vi "Save Configuration Settings to XML.vi"(8 "error in (no error)":errorcluster, 11 "User Configuration":T1={"Hardware Configuration"={"HW Refnum <Replace Me>"="", "Signal Type <Replace Me>"=enum."Sine Wave"}, "Analysis Configuration"={"Statistics"=TRUE}, "New Data Behavior"=enum."Replace"}) -> (0 "error out":errorcluster)   [LabVIEW 2012]
doc: "Saves the user-specified configuration data to an XML file. This is used to remember settings between executions."
uses:
  controls/User Specified Data.ctl
  controls/HW Configuration.ctl
  controls/Simulated Signal Type.ctl
  controls/Analysis Configuration.ctl
  controls/New Data Behavior.ctl
  <vilib>/Utility/xml.llb/Write to XML File(string).vi
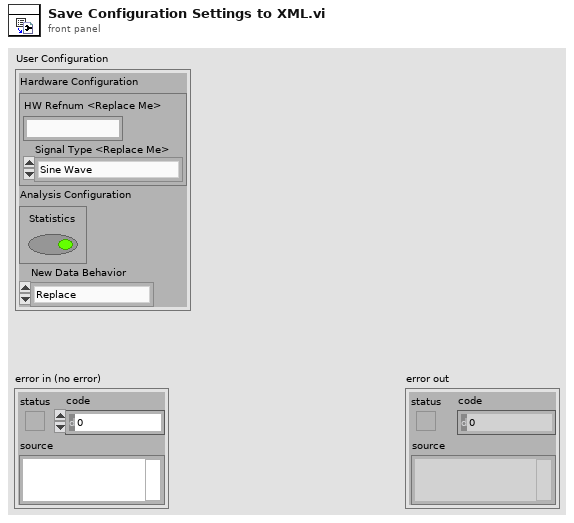
[diagram p1: front panel]
types:
  T1 = typedef "User Specified Data.ctl" = cluster{"Hardware Configuration":T2, "Analysis Configuration":T4, "New Data Behavior":T5}
  T2 = typedef "HW Configuration.ctl" = cluster{"HW Refnum <Replace Me>":string, "Signal Type <Replace Me>":T3}
  T3 = typedef "Simulated Signal Type.ctl" = enum16{"Sine Wave", "Square Wave"}
  T4 = typedef "Analysis Configuration.ctl" = cluster{"Statistics":bool}
  T5 = typedef "New Data Behavior.ctl" = enum16{"Replace", "Overlay", "Append"}
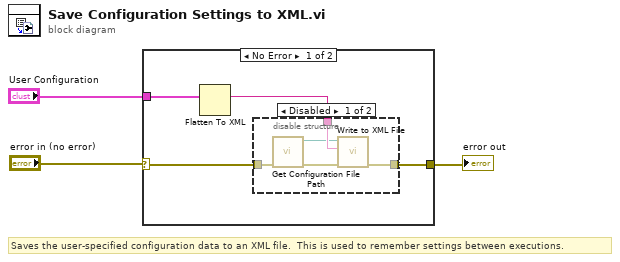
[diagram p0: block diagram]
diagram:
  # "Saves the user-specified configuration data to an XML file.  This is used to remember settings between executions."
  n1 = case shown="No Error" "error in (no error)" {
    selector: "error in (no error)" -> [w4 w14]
    tunnel: [w5 w14] -> w2
    tunnel: "User Configuration" -> [w7 _]
    frame No Error {
      n2 = Flatten To XML(anything=w7) -> (xml string=w6:string)
      n3 = disable-structure shown="Disabled" {
        disable-tunnel: w6 -> [w12 _]
        disable-tunnel: [w11 w13] -> w5
        disable-tunnel: w4 -> [w9 w13]
        frame Disabled {
          n4 = call "Get Configuration File Path.vi"("error in (no error)"=w9) -> ("error out"=w8:errorcluster, "XML File Path"=w10:path)  [unwired: 9 in]
          n5 = call-poly <vilib>:"Write to XML File.vi"("error in (no error)"=w8, "XML Input"=w12, "XML File Path"=w10) -> ("error out"=w11:errorcluster)  [unwired: 6 in, 2 out]
        }
        frame Enabled {
          # "Disabled to prevent\nerror saving to Program\nFiles"
        }
      }
    }
    frame Error {
    }
  }
  "error out" <- w2
